vi "create_dataset.vi"() -> ()   [LabVIEW 2024]
uses:
  controls/class.ctl
  controls/cluster.ctl
  <vilib>/vision/Image Controls.llb/IMAQ Image.ctl
  <vilib>/vision/NI_Vision_Development_Module.lvlib
panel:
  in  "Redo":bool
  in  "Undo":bool
  in  "Stop":bool
  in  "Help":bool
  in  "Next":bool
  in  "Previous":bool
  out "Number of features:":dbl
  in  "Feature Type:":T1 items=["weld", "corrugation"]
  in  "Change Directory":bool
  out "Current Image name":string
  in  "Database Directory:":path=path "C:/Users/Naomi Tan/Documents/Gillette/FACE/02 - Code/FACE_software/images/test/ST100242_CAMFACE_LOCGLICR_RN3147_SHV3Post_POSleft.jpg"
  in  "Tab Control":enum32{"Setup", "Create"}(tab)
  in  "Dataset Directory:":path=path "C:/Users/J Gordon/Documents/Create Dataset/images"
  in  "Image Directory/File:":path=path "C:/Users/J Gordon/Documents/Create Dataset/images/test"
  in  "Start":bool
  out "of":i32
  out "Image":i32
  out "Image":T2(plugin-control)
  out "Zoom Window":T2(plugin-control)
  # "Create Custom\nDataset"
  # "Select Directories"
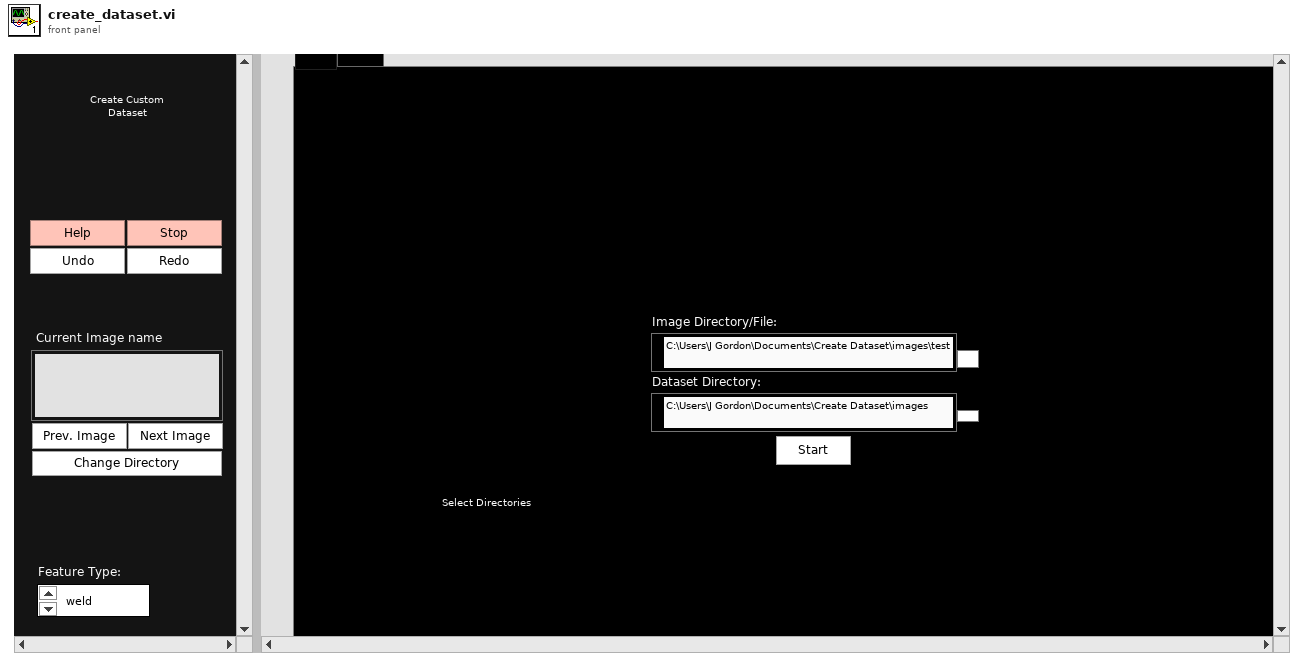
[diagram p1: front panel]
types:
  T1 = typedef "Class.ctl" = u16
  T2 = typedef "IMAQ Image.ctl" = refnum<image>
  T3 = enum8{"Enabled", "Disabled", "Disabled and Grayed Out"}
  T4 = cluster{"[0]":dbl, "[1]":dbl, "[2]":dbl, "[3]":dbl}[]
  T5 = typedef "cluster.ctl" = cluster{"Image path":path, "Image path array":path[], "Image index":u32, "Dataset Directory:":path, "Exists":bool, "classes":string[], "bboxes":cluster{"[0]":dbl, "[1]":dbl, "[2]":dbl, "[3]":dbl}[], "n":dbl, "Image":T2, "Image name":string, "classes history":string[], "bboxes":cluster{"[0]":dbl, "[1]":dbl, "[2]":dbl, "[3]":dbl}[], "Model Path:":path, "Classes Path:":path, "scores":dbl[], "Confidence":dbl}
  T6 = cluster{"[0]":i32, "[1]":i32, "[2]":i32, "[3]":i32}[]
  T7 = typedef "Image Type" = u32
  T8 = cluster{"Global Rectangle":i32[], "Contours":cluster{"Contour Type":u32, "ROI Type":u32, "Points":i32[]}[]}
  T9 = cluster{"Numeric Control":dbl, "Numeric Control":dbl, "width":dbl, "height":dbl}
  T10 = cluster{"Numeric Control":dbl, "Numeric Control":dbl, "width":dbl, "height":dbl}[]
  T11 = cluster{"[0]":dbl, "[1]":dbl, "[2]":dbl, "[3]":dbl}
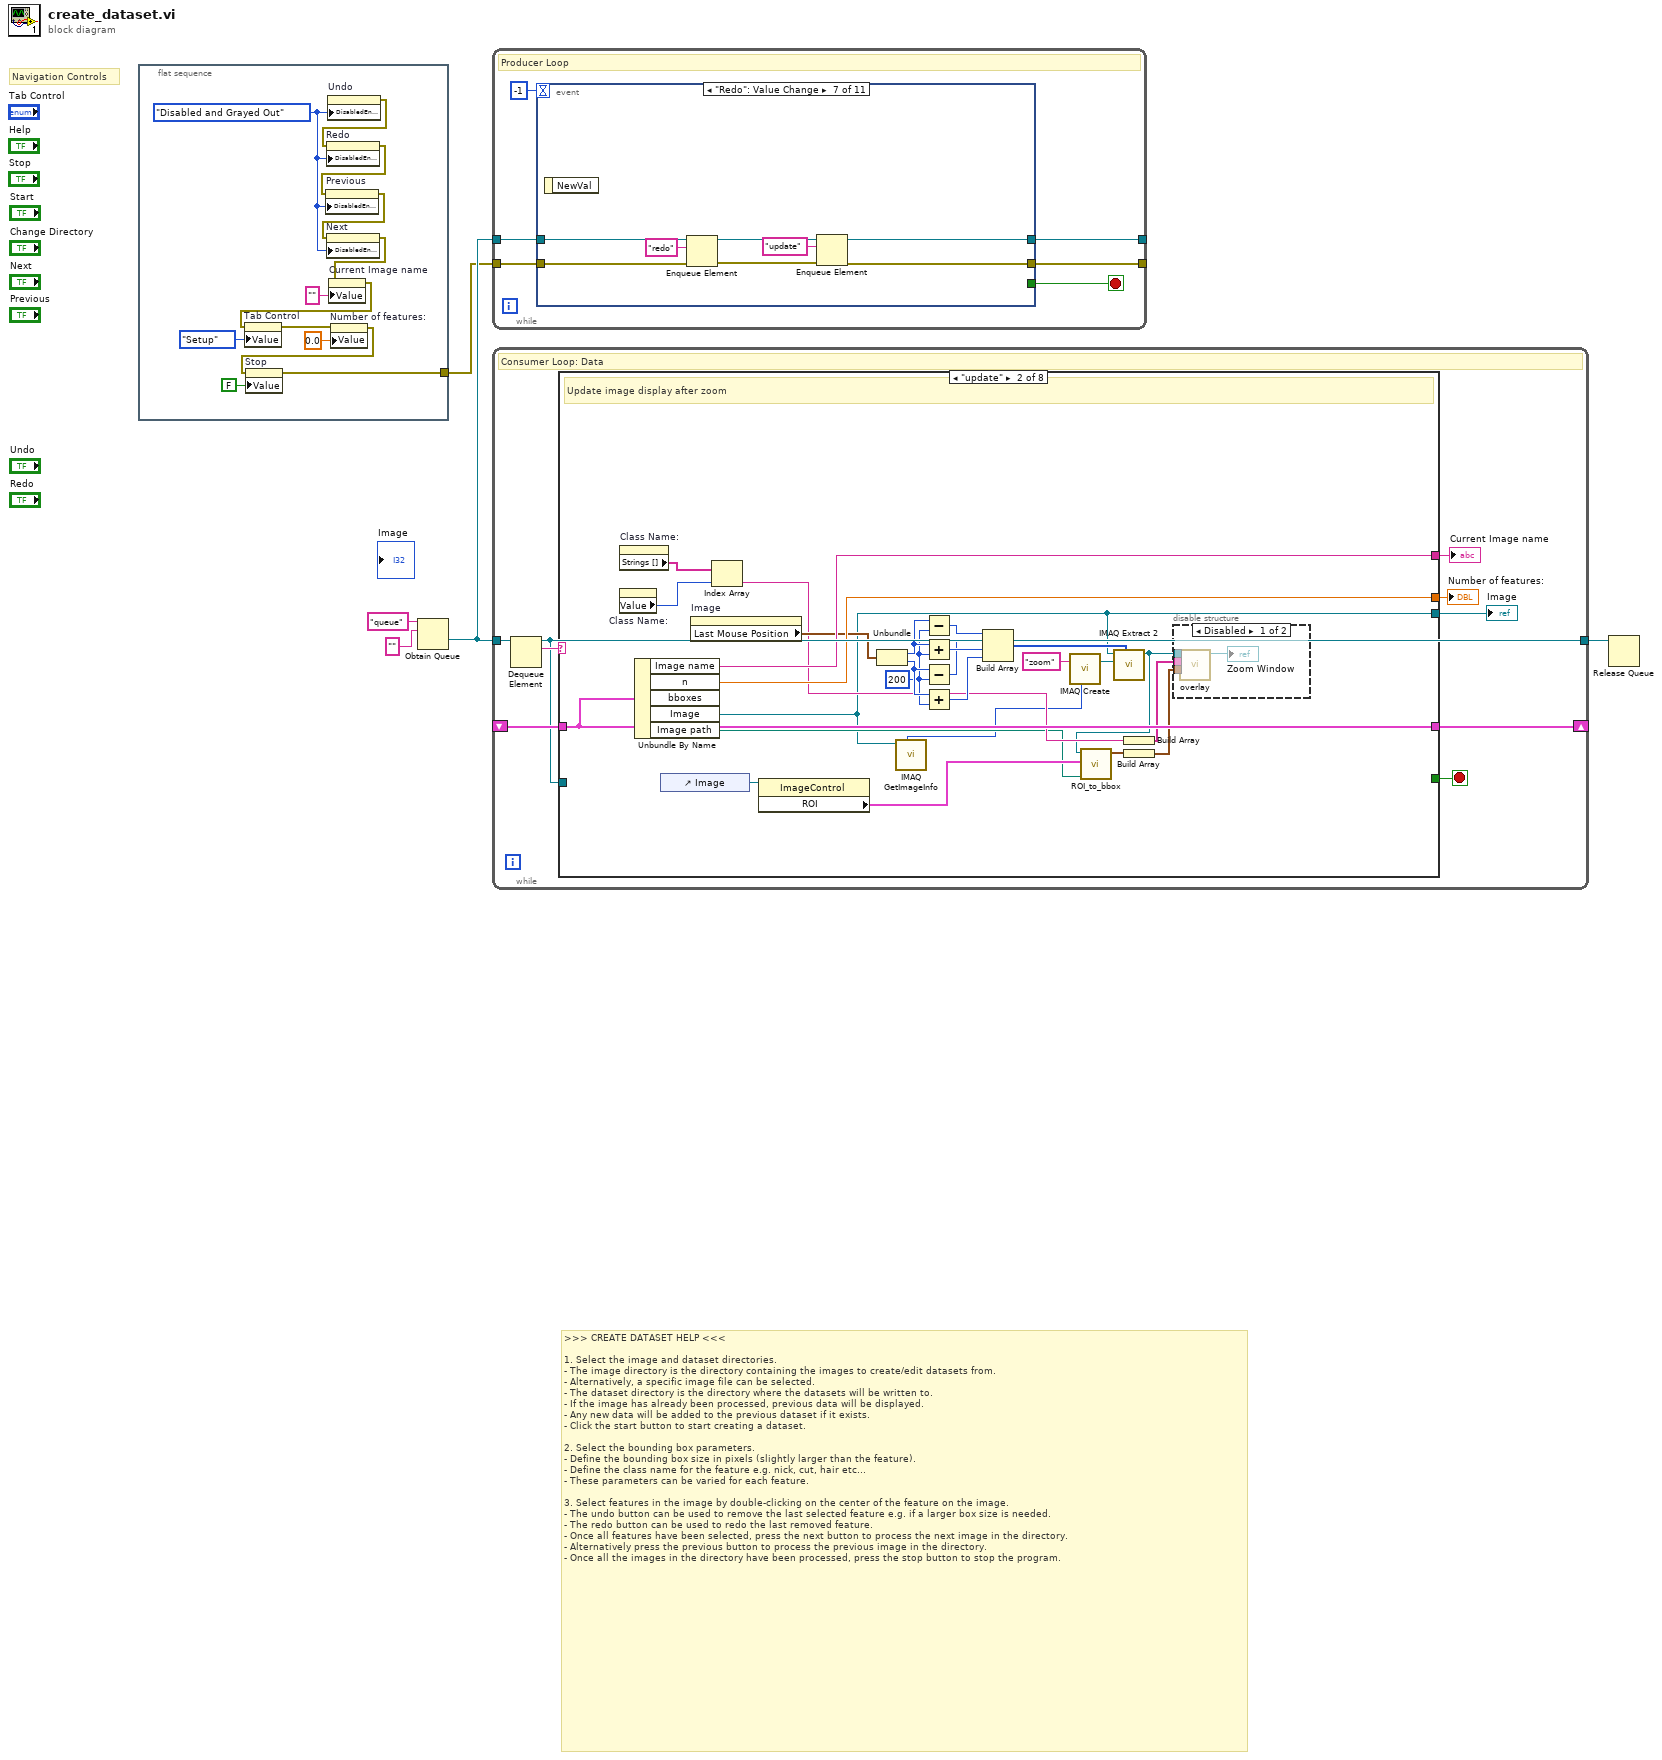
[diagram p0: block diagram]
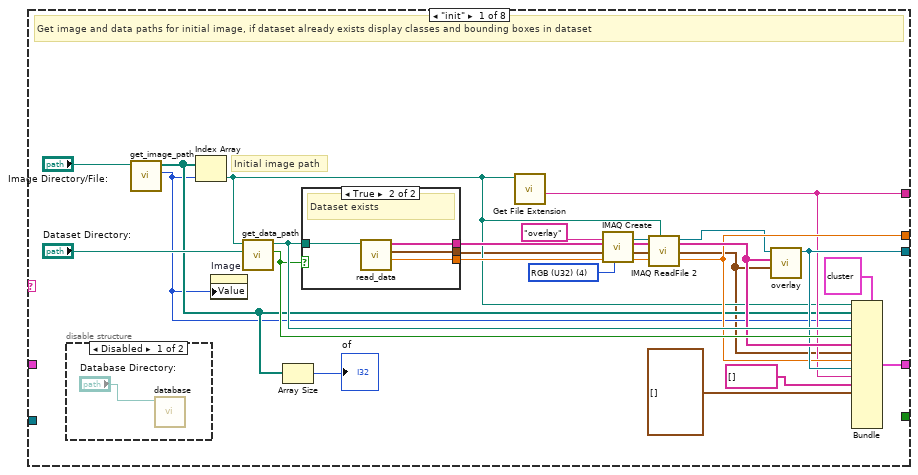
[diagram p2: hidden frame]
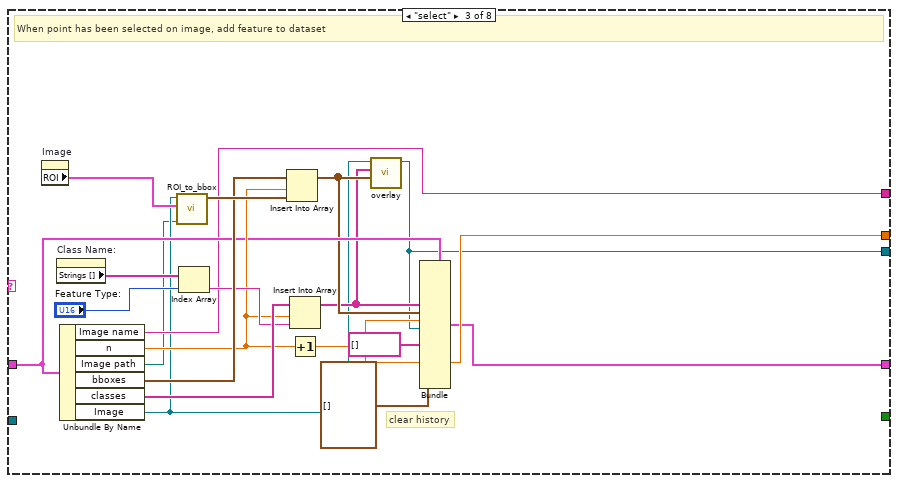
[diagram p6: hidden frame]
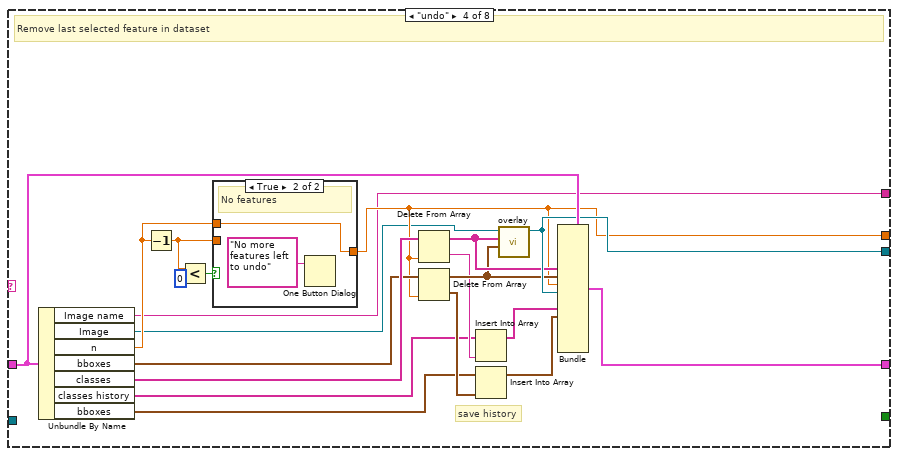
[diagram p7: hidden frame]
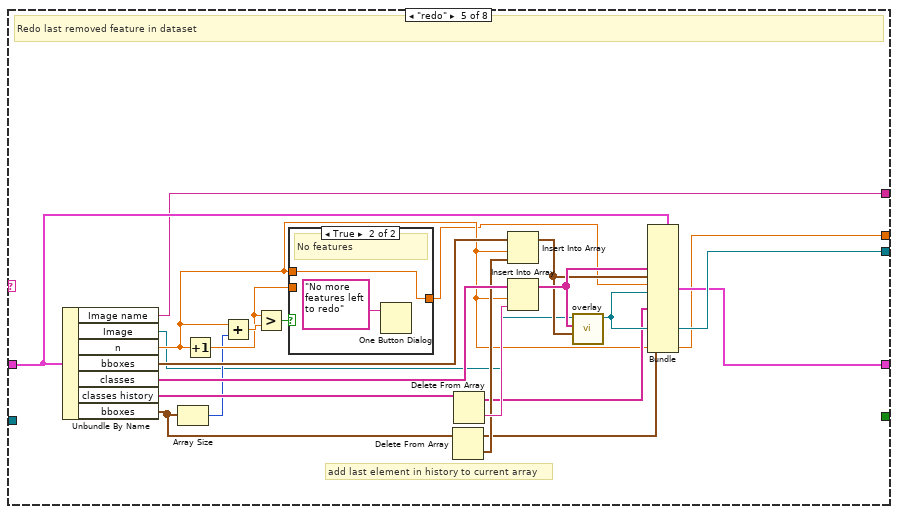
[diagram p9: hidden frame]
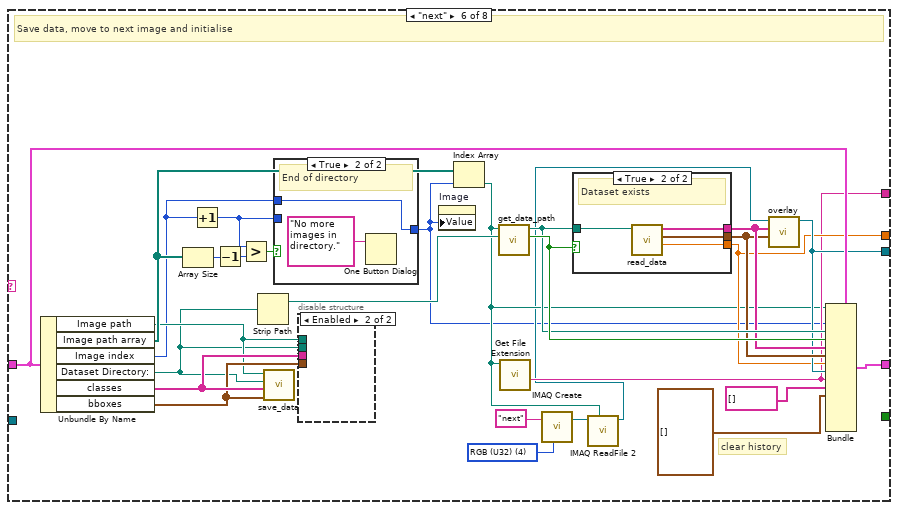
[diagram p11: hidden frame]
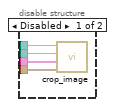
[diagram p12: hidden frame]
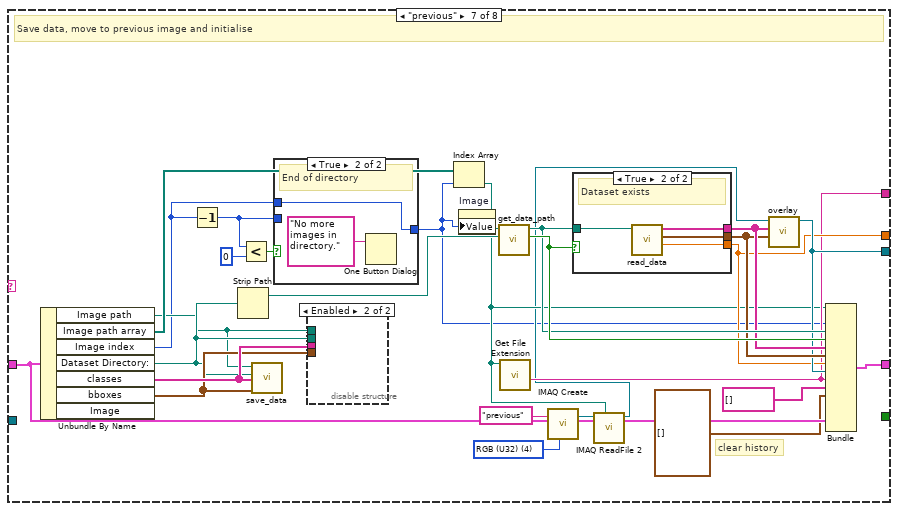
[diagram p15: hidden frame]
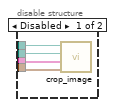
[diagram p16: hidden frame]
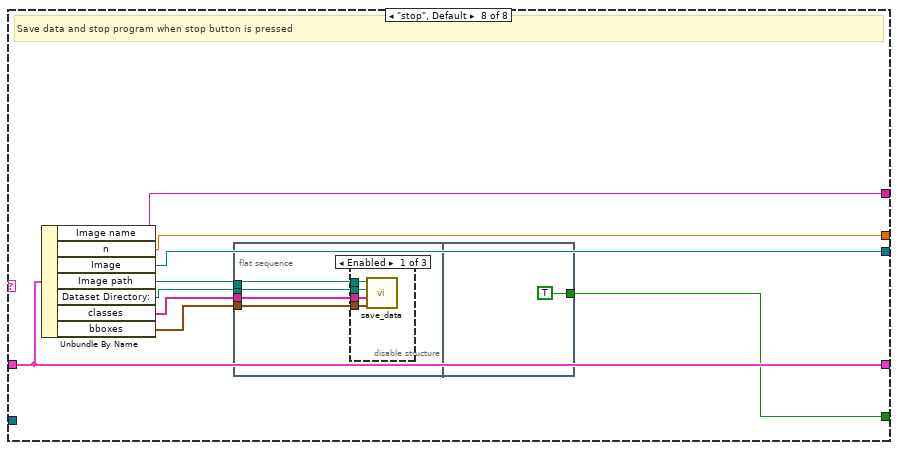
[diagram p19: hidden frame]
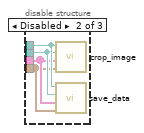
[diagram p20: hidden frame]
diagram:
  # ">>> CREATE DATASET HELP <<<\n\n1. Select the image and dataset directories.\n- The image directory is the directory containing the images to create/edit datasets from.\n- Alternatively, a specific image file can be selected.\n- The dataset directory is the directory where the datasets will be written to.\n- If the image has already been processed, previous data will be displayed.\n- Any new data will be added to the previous dataset if it exists.\n- Click the start button to start creating a dataset.\n\n2. Select the bounding box parameters.\n- Define the bounding box size in pixels (slightly larger than the feature).\n- Define the class name for the feature e.g. nick, cut, hair etc...\n- These parameters can be varied for each feature.\n\n3. Select features in the image by double-clicking on the center of the feature on the image.\n- The undo button can be used to remove the last selected feature e.g. if a larger box size is needed.\n- The redo button can be used to redo the last removed feature.\n- Once all features have been selected, press the next button to process the next image in the directory.\n- Alternatively press the previous button to process the previous image in the directory.\n- Once all the images in the directory have been processed, press the stop button to stop the program."
  # "Navigation Controls"
  n1 = flat-sequence {
    tunnel: [w6] -> w2
    frame #0 {
      w14 = T3."Disabled and Grayed Out" ("Disabled")
      n2 = property on="Undo" class="Bool"("DisabledEnum"=w14) -> (error out=w13:errorcluster)  [unwired: 2 in, 1 out]
      n3 = property on="Redo" class="Bool"(error in=w13, "DisabledEnum"=w14) -> (error out=w12:errorcluster)  [unwired: 1 in, 1 out]
      n4 = property on="Previous" class="Bool"(error in=w12, "DisabledEnum"=w14) -> (error out=w11:errorcluster)  [unwired: 1 in, 1 out]
      n5 = property on="Next" class="Bool"(error in=w11, "DisabledEnum"=w14) -> (error out=w10:errorcluster)  [unwired: 1 in, 1 out]
      n6 = property on="Current Image name" class="Str"(error in=w10, "Value"="" ("Image name:")) -> (error out=w9:errorcluster)  [unwired: 1 in, 1 out]
      n7 = property on="Tab Control" class="TabCtl (strict)"(error in=w9, "Value"=enum32{"Setup", "Create"}."Setup" ("Tab Control")) -> (error out=w8:errorcluster)  [unwired: 1 in, 1 out]
      n8 = property on="Number of features:" class="DigNum (strict)"(error in=w8, "Value"=0.0 ("Number of features:")) -> (error out=w7:errorcluster)  [unwired: 1 in, 1 out]
      n9 = property on="Stop" class="Bool (strict)"(error in=w7, "Value"=FALSE ("Stop Button")) -> (error out=w6:errorcluster)  [unwired: 1 in, 1 out]
    }
  }
  n10 = Obtain Queue(name (unnamed)="queue", element data type="" ("name (unnamed)")) -> (queue out=w3:refnum<queue>)  [unwired: 3 in, 2 out]
  n11 = while {
    tunnel: w3 -> [w23]
    tunnel: [w22] -> _
    tunnel: [w21] -> _
    tunnel: w2 -> [w20]
    stop <- w24 stop-if-true
    # "Producer Loop"
    n12 = event shown="[6] \"Redo\": Value Change" {
      selector: _ -> [_ _ _ _ _ _ _ _ _ _ _]
      dyn-events: _ -> [_ _ _ _ _ _ _ _ _ _ _]
      timeout: -1 -> [_ _ _ _ _ _ _ _ _ _ _]
      tunnel: w23 -> [w27 w33 w41 w59 w64 w99 w107 w114 w122 w125 w130]
      tunnel: [w27 w31 w42 w59 w63 w93 w103 w111 w120 w125 w129] -> w22
      tunnel: [_ TRUE _ _ _ _ _ _ _ _ _] -> w24
      tunnel: [w25 w29 w40 w56 w62 w92 w102 w109 w119 w124 w127] -> w21
      tunnel: w20 -> [w25 w28 w34 w56 w61 w97 w105 w108 w116 w124 w128]
      event "Help": Value Change {
        n13 = event-data() -> ()  [unwired: 1 in, 1 out]
        n14 = One Button Dialog(message="                                                                 >>> CREATE DATASET HELP <<<\n\n1. Select the image and dataset directories.\n- The image directory is the directory containing the images to create/edit datasets from.\n- Alternatively, a specific image file can be selected.\n- The dataset directory is the directory where the datasets will be written to.\n- If the image has already been processed, previous data will be displayed.\n- Any new data will be added to the previous dataset if it exists.\n- Click the start button to start creating a dataset.\n\n2. Select the bounding box parameters.\n- Define the bounding box size in pixels (slightly larger than the feature).\n- Define the class name for the feature e.g. nick, cut, hair etc...\n- These parameters can be varied for each feature.\n\n3. Select features in the image by double-clicking on the center of the feature on the image.\n- The undo button can be used to remove the last selected feature e.g. if a larger box size is needed.\n- The redo button can be used to redo the last removed feature.\n- Once all features have been selected, press the next button to process the next image in the directory.\n- Alternatively press the previous button to process the previous image in the directory.\n- Once all the images in the directory have been processed, press the stop button to stop the program.") -> ()  [unwired: 1 in, 1 out]
      }
      event "Stop": Value Change {
        n15 = event-data() -> ()  [unwired: 1 in, 1 out]
        n16 = Enqueue Element(queue=w33, element="stop" ("name (unnamed)"), error in (no error)=w28) -> (queue out=w31:refnum<queue>, error out=w29:errorcluster)  [unwired: 1 in, 1 out]
      }
      event "Start": Value Change {
        n17 = event-data() -> ()  [unwired: 1 in, 1 out]
        n18 = property on="Image Directory/File:" class="Path"() -> ("Value"=w36:path)  [unwired: 2 in, 2 out]
        n19 = property on="Dataset Directory:" class="Path"() -> ("Value"=w37:path)  [unwired: 2 in, 2 out]
        n20 = call <vilib>:"Check if File or Folder Exists.vi"("path"=w36) -> ("file or folder exists?"=w39:bool)  [unwired: 8 in, 2 out]
        n21 = call <vilib>:"Check if File or Folder Exists.vi"("path"=w37) -> ("file or folder exists?"=w38:bool)  [unwired: 8 in, 2 out]
        n22 = And(x=w39, y=w38) -> (x .and. y?=w35:bool)
        n23 = case shown="True" w35 {
          tunnel: [w45 w50] -> w42
          tunnel: w41 -> [w45 w54]
          tunnel: [w43 w47] -> w40
          tunnel: w34 -> [w43 w46]
          frame False {
            # "Directories don't exist"
            n24 = One Button Dialog(message="Image or dataset directory does not exist, please select another directory") -> ()  [unwired: 1 in, 1 out]
          }
          frame True {
            w52 = T3."Enabled" ("Disabled")
            # "Directories exist"
            n25 = Enqueue Element(queue=w54, element="init", error in (no error)=w46) -> (queue out=w49:refnum<queue>, error out=w48:errorcluster)  [unwired: 1 in, 1 out]
            n26 = property on="Tab Control" class="TabCtl (strict)"("Value"=enum32{"Setup", "Create"}."Create" ("Tab Control")) -> ()  [unwired: 2 in, 2 out]
            n27 = property on="Redo" class="Bool"("DisabledEnum"=w52) -> ()  [unwired: 2 in, 2 out]
            n28 = property on="Previous" class="Bool"("DisabledEnum"=w52) -> ()  [unwired: 2 in, 2 out]
            n29 = property on="Next" class="Bool"("DisabledEnum"=w52) -> ()  [unwired: 2 in, 2 out]
            n30 = Enqueue Element(queue=w49, element="update", error in (no error)=w48) -> (queue out=w50:refnum<queue>, error out=w47:errorcluster)  [unwired: 1 in, 1 out]
            n31 = property on="Undo" class="Bool"("DisabledEnum"=w52) -> ()  [unwired: 2 in, 2 out]
          }
        }
      }
      event "Change Directory": Value Change {
        w57 = T3."Disabled and Grayed Out" ("Disabled")
        n32 = event-data() -> ()  [unwired: 1 in, 1 out]
        n33 = property on="Tab Control" class="TabCtl (strict)"("Value"=enum32{"Setup", "Create"}."Setup" ("Tab Control")) -> ()  [unwired: 2 in, 2 out]
        n34 = property on="Undo" class="Bool"("DisabledEnum"=w57) -> ()  [unwired: 2 in, 2 out]
        n35 = property on="Redo" class="Bool"("DisabledEnum"=w57) -> ()  [unwired: 2 in, 2 out]
        n36 = property on="Previous" class="Bool"("DisabledEnum"=w57) -> ()  [unwired: 2 in, 2 out]
        n37 = property on="Next" class="Bool"("DisabledEnum"=w57) -> ()  [unwired: 2 in, 2 out]
      }
      event "Image": Mouse Up {
        n38 = event-data() -> ()  [unwired: 1 in, 1 out]
        n39 = disable-structure shown="Enabled" {
          disable-tunnel: w64 -> [w69 w84 _]
          disable-tunnel: [w68 w83 _] -> w63
          disable-tunnel: [w67 w82 _] -> w62
          disable-tunnel: TRUE ("Double Click") -> [w66 w81 _]
          disable-tunnel: w61 -> [w65 w80 _]
          frame Enabled {
            n40 = case shown="True" w66 {
              tunnel: w69 -> [w71 w78]
              tunnel: [w71 w74] -> w68
              tunnel: [w70 w72] -> w67
              tunnel: w65 -> [w70 w77]
              frame False {
              }
              frame True {
                n41 = Enqueue Element(queue=w78, element="select" ("name (unnamed)"), error in (no error)=w77) -> (queue out=w75:refnum<queue>, error out=w73:errorcluster)  [unwired: 1 in, 1 out]
                n42 = Enqueue Element(queue=w75, element="update" ("name (unnamed)"), error in (no error)=w73) -> (queue out=w74:refnum<queue>, error out=w72:errorcluster)  [unwired: 1 in, 1 out]
              }
            }
          }
          frame Disabled {
            n43 = case shown="True" w81 {
              tunnel: w84 -> [w86 w90]
              tunnel: [w86 w88] -> w83
              tunnel: [w85 w87] -> w82
              tunnel: w80 -> [w85 w89]
              frame False {
              }
              frame True {
                n44 = Enqueue Element(queue=w90, element="box" ("name (unnamed)"), error in (no error)=w89) -> (queue out=w88:refnum<queue>, error out=w87:errorcluster)  [unwired: 1 in, 1 out]
              }
            }
          }
          frame Disabled {
          }
        }
      }
      event "Undo": Value Change {
        n45 = event-data() -> ()  [unwired: 1 in, 1 out]
        n46 = Enqueue Element(queue=w99, element="undo", error in (no error)=w97) -> (queue out=w95:refnum<queue>, error out=w94:errorcluster)  [unwired: 1 in, 1 out]
        n47 = Enqueue Element(queue=w95, element="update", error in (no error)=w94) -> (queue out=w93:refnum<queue>, error out=w92:errorcluster)  [unwired: 1 in, 1 out]
      }
      event "Redo": Value Change {
        n48 = event-data() -> ()  [unwired: 1 in, 1 out]
        n49 = Enqueue Element(queue=w107, element="redo", error in (no error)=w105) -> (queue out=w100:refnum<queue>, error out=w101:errorcluster)  [unwired: 1 in, 1 out]
        n50 = Enqueue Element(queue=w100, element="update", error in (no error)=w101) -> (queue out=w103:refnum<queue>, error out=w102:errorcluster)  [unwired: 1 in, 1 out]
      }
      event "Next": Value Change {
        n51 = event-data() -> ()  [unwired: 1 in, 1 out]
        n52 = Enqueue Element(queue=w114, element="next", error in (no error)=w108) -> (queue out=w112:refnum<queue>, error out=w110:errorcluster)  [unwired: 1 in, 1 out]
        n53 = Enqueue Element(queue=w112, element="update", error in (no error)=w110) -> (queue out=w111:refnum<queue>, error out=w109:errorcluster)  [unwired: 1 in, 1 out]
      }
      event "Previous": Value Change {
        n54 = event-data() -> ()  [unwired: 1 in, 1 out]
        n55 = Enqueue Element(queue=w122, element="previous", error in (no error)=w116) -> (queue out=w117:refnum<queue>, error out=w118:errorcluster)  [unwired: 1 in, 1 out]
        n56 = Enqueue Element(queue=w117, element="update", error in (no error)=w118) -> (queue out=w120:refnum<queue>, error out=w119:errorcluster)  [unwired: 1 in, 1 out]
      }
      event Timeout {
        n57 = event-data() -> ()  [unwired: 1 in, 1 out]
      }
      event "Image": Mouse Move {
        n58 = event-data() -> ()  [unwired: 1 in, 5 out]
        n59 = Enqueue Element(queue=w130, element="update", error in (no error)=w128) -> (queue out=w129:refnum<queue>, error out=w127:errorcluster)  [unwired: 1 in, 1 out]
      }
    }
  }
  n60 = while {
    tunnel: w3 -> [w139]
    tunnel: [w131] -> w1
    shift-right: [w135] -> _
    shift-left: _ -> [w133]
    stop <- w137 stop-if-true
    # "Consumer Loop: Data"
    n61 = Dequeue Element(queue=w139) -> (queue out=w131:refnum<queue>, element=w138:string)  [unwired: 2 in, 2 out]
    n62 = case shown="\"update\"" w138 {
      tunnel: [w155 w191 w204 w224 w240 w277 w315 w343] -> w136
      tunnel: [_ _ _ _ _ _ _ w339] -> w137
      tunnel: [w156 w167 w202 w233 w257 w278 w316 w341] -> w132
      tunnel: [w157 w190 w203 w228 w252 w284 w324 w347] -> w135
      tunnel: [w154 w189 w200 w220 w251 w276 w314 w340] -> w134
      tunnel: w133 -> [_ w190 w207 w234 w258 w285 w325 w347]
      tunnel: w131 -> [_ _ _ _ _ _ _ _]
      frame "init" {
        w147 = T7 4 items=["Grayscale (U8)", "Grayscale (I16)", "Grayscale (SGL)", "Complex (CSG)", "RGB (U32)", "HSL (U32)", "RGB (U64)", "Grayscale (U16)"] ("Image Type")
        # "Initial image path"
        # "Get image and data paths for initial image, if dataset already exists display classes and bounding boxes in dataset"
        n63 = disable-structure shown="Disabled" {
          frame Disabled {
            n64 = call "database.vi"("db file"="Database Directory:") -> ()  [unwired: 9 in, 2 out]
          }
          frame Enabled {
          }
        }
        n65 = call "get_image_path.vi"("Image directory/path"="Image Directory/File:") -> ("Init image index"=w142:u32, "Image path array"=w144:path[])  [unwired: 9 in]
        n66 = Index Array(array=w144, index=w142) -> (element=w146:path)
        n67 = property on="Image" class="DigNum (strict)"("Value"=w142) -> ()  [unwired: 2 in, 2 out]
        n68 = call "get_data_path.vi"("Dataset directory"="Dataset Directory:", "Image path"=w146) -> ("Exists"=w159:bool, "Dataset path"=w160:path)  [unwired: 8 in]
        n69 = Array Size(array=w144) -> (size(s)=→"of":i32)
        n70 = case shown="True" w159 {
          tunnel: w160 -> [_ w162]
          tunnel: [_ w165] -> w141
          tunnel: [_ w164] -> w155
          tunnel: [_ w163] -> w158
          frame False {
            # "Dataset doesn't exist"
          }
          frame True {
            # "Dataset exists"
            n71 = call "read_data.vi"("Data path"=w162) -> ("n"=w164:dbl, "bboxes"=w165:T4, "classes"=w163:string[])  [unwired: 7 in, 1 out]
          }
        }
        n72 = call <vilib>:"Get File Extension.vi"("file"=w146) -> ("filename without extension"=w154:string)  [unwired: 6 in, 4 out]
        n73 = call "IMAQ Create"("Image Name"="overlay", "Image Type"=w147) -> ("New Image"=w148:T2)  [unwired: 3 in, 1 out]
        n74 = call "IMAQ ReadFile 2"("File Path"=w146, "Image"=w148) -> ("Image Out"=w145:T2)  [unwired: 5 in, 4 out]
        n75 = call "overlay.vi"("Image in"=w145, "classes"=w158, "bboxes"=w141) -> ("Image"=w156:T2)  [unwired: 7 in]
        n76 = Bundle(cluster=T5 {"Image path"=path "", "Image path array"=[], "Image index"=0, "Dataset Directory:"=path "", "Exists"=FALSE, "classes"=[], "bboxes"=[], "n"=0.0, "Image"=refnum, "Image name"="", "classes history"=[], "bboxes"=[], "Model Path:"=path "", "Classes Path:"=path "", "scores"=[], "Confidence"=0.0}, "Image path"=w146, "Image path array"=w144, "Image index"=w142, "Dataset Directory:"=w160, "Exists"=w159, "classes"=w158, "bboxes"=w141, "n"=w155, "Image"=w156, "Image name"=w154, "classes history"=string[] [], "bboxes"=T4 []) -> (w157:T5)  [unwired: 4 in]
      }
      frame "update" {
        w180 = 200 ("y")
        # "Update image display after zoom"
        n77 = property on="Class Name:" class="Ring (strict)"() -> ("Strings []"=w175:string[])  [unwired: 2 in, 2 out]
        n78 = property on="Class Name:" class="Ring (strict)"() -> ("Value"=w176:T1)  [unwired: 2 in, 2 out]
        n79 = Unbundle By Name(w190) -> ("Image name"=w189:string, "n"=w191:dbl, "Image"=w167:T2, "Image path"=w168:path)  [unwired: 1 out]
        n80 = control-ref of="Image"() -> (w170:refnum<vi>)
        n81 = property on="Image" class="ImageControl"() -> ("Last Mouse Position"=w185:cluster{"X":i32, "Y":i32})  [unwired: 2 in, 2 out]
        n82 = Index Array(array=w175, index=w176) -> (element=w173:string)
        n83 = property class="ImageControl"(reference=w170) -> ("ROI"=w169:T8)  [unwired: 1 in, 2 out]
        n84 = Unbundle(w185) -> ("X"=w182:i32, "Y"=w181:i32)
        n85 = call "IMAQ GetImageInfo"("Image"=w167) -> ("Image Type"=w166:T7)  [unwired: 3 in, 7 out]
        n86 = Subtract(x=w182, y=w180) -> (x-y=w179:i32)
        n87 = Add(x=w182, y=w180) -> (x+y=w186:i32)
        n88 = Subtract(x=w181, y=w180) -> (x-y=w178:i32)
        n89 = Add(x=w181, y=w180) -> (x+y=w187:i32)
        n90 = Build Array(w179, w178, w186, w187) -> (w188:i32[])
        n91 = call "IMAQ Create"("Image Name"="zoom", "Image Type"=w166) -> ("New Image"=w184:T2)  [unwired: 3 in, 1 out]
        n92 = call "IMAQ Extract 2"("Optional Rectangle"=w188, "Image Dst"=w184, "Image Src"=w167) -> ("Image Dst Out"=w171:T2)  [unwired: 7 in, 1 out]
        n93 = call "ROI_to_bbox.vi"("Image path"=w168, "ROI"=w169, "Image in"=w171) -> ("bbox"=w174:T9)  [unwired: 8 in]
        n94 = Build Array(w173) -> (w172:string[])
        n95 = Build Array(w174) -> (w177:T10)
        n96 = disable-structure shown="Disabled" {
          disable-tunnel: w177 -> [w195 _]
          disable-tunnel: w172 -> [w194 _]
          disable-tunnel: w171 -> [w192 _]
          frame Disabled {
            n97 = call "overlay.vi"("Image in"=w192, "classes"=w194, "bboxes"=w195) -> ("Image"=→"Zoom Window":T2)  [unwired: 7 in]
          }
          frame Enabled {
          }
        }
      }
      frame "select" {
        # "clear history"
        # "When point has been selected on image, add feature to dataset"
        n98 = property on="Image" class="ImageControl"() -> ("ROI"=w214:T8)  [unwired: 2 in, 2 out]
        n99 = property on="Class Name:" class="Ring (strict)"() -> ("Strings []"=w212:string[])  [unwired: 2 in, 2 out]
        n100 = Unbundle By Name(w207) -> ("Image name"=w200:string, "n"=w208:dbl, "Image path"=w196:path, "bboxes"=w211:T4, "classes"=w210:string[], "Image"=w197:T2)
        n101 = call "ROI_to_bbox.vi"("Image path"=w196, "ROI"=w214, "Image in"=w197) -> ("bbox"=w213:T9)  [unwired: 8 in]
        n102 = Index Array(array=w212, index="Feature Type:") -> (element=w209:string)
        n103 = Insert Into Array(array=w211, index=w208, new element=w213) -> (w206:T4)
        n104 = Insert Into Array(array=w210, index=w208, new element=w209) -> (w205:string[])
        n105 = Increment(x=w208) -> (x+1=w204:dbl)
        n106 = call "overlay.vi"("Image in"=w197, "classes"=w205, "bboxes"=w206) -> ("Image"=w202:T2)  [unwired: 7 in]
        n107 = Bundle(cluster=w207, "classes"=w205, "bboxes"=w206, "n"=w204, "Image"=w202, "classes history"=string[] [], "bboxes"=T6 [] ("bboxes history")) -> (w203:T5)  [unwired: 10 in]
      }
      frame "undo" {
        # "save history"
        # "Remove last selected feature in dataset"
        n108 = Unbundle By Name(w234) -> ("Image name"=w220:string, "Image"=w215:T2, "n"=w221:dbl, "bboxes"=w231:T4, "classes"=w232:string[], "classes history"=w219:string[], "bboxes"=w218:T4)
        n109 = Decrement(x=w221) -> (x-1=w226:dbl)
        n110 = Less?(x=w226, y=u32 0) -> (x < y?=w227:bool)
        n111 = case shown="True" w227 {
          tunnel: w226 -> [w235 _]
          tunnel: [w235 w236] -> w224
          tunnel: w221 -> [_ w236]
          frame False {
            # "Index in range"
          }
          frame True {
            # "No features"
            n112 = One Button Dialog(message="No more features left to undo") -> ()  [unwired: 1 in, 1 out]
          }
        }
        n113 = Delete From Array(array=w232, index=w224) -> (deleted portion=w223:string, array with subset deleted=w230:string[])  [unwired: 1 in]
        n114 = Delete From Array(array=w231, index=w224) -> (deleted portion=w222:T11, array with subset deleted=w229:T4)  [unwired: 1 in]
        n115 = Insert Into Array(array=w219, new element=w223) -> (w217:string[])  [unwired: 1 in]
        n116 = Insert Into Array(array=w218, new element=w222) -> (w216:T4)  [unwired: 1 in]
        n117 = call "overlay.vi"("Image in"=w215, "classes"=w230, "bboxes"=w229) -> ("Image"=w233:T2)  [unwired: 7 in]
        n118 = Bundle(cluster=w234, "classes"=w230, "bboxes"=w229, "n"=w224, "Image"=w233, "classes history"=w217, "bboxes"=w216) -> (w228:T5)  [unwired: 10 in]
      }
      frame "redo" {
        # "add last element in history to current array"
        # "Redo last removed feature in dataset"
        n119 = Unbundle By Name(w258) -> ("Image name"=w251:string, "Image"=w238:T2, "n"=w240:dbl, "bboxes"=w255:T4, "classes"=w256:string[], "classes history"=w250:string[], "bboxes"=w242:T4)
        n120 = Array Size(array=w242) -> (size(s)=w241:i32)
        n121 = Increment(x=w240) -> (x+1=w243:dbl)
        n122 = Add(x=w240, y=w241) -> (x+y=w245:dbl)
        n123 = Greater?(x=w243, y=w245) -> (0:w244:bool)
        n124 = case shown="True" w244 {
          tunnel: w243 -> [w259 _]
          tunnel: [w259 w260] -> w239
          tunnel: w240 -> [_ w260]
          frame False {
            # "Index in range"
          }
          frame True {
            # "No features"
            n125 = One Button Dialog(message="No more features left to redo") -> ()  [unwired: 1 in, 1 out]
          }
        }
        n126 = Delete From Array(array=w242) -> (deleted portion=w248:T11, array with subset deleted=w246:T4)  [unwired: 2 in]
        n127 = Delete From Array(array=w250) -> (deleted portion=w249:string, array with subset deleted=w247:string[])  [unwired: 2 in]
        n128 = Insert Into Array(array=w255, index=w240, new element=w248) -> (w253:T4)
        n129 = Insert Into Array(array=w256, index=w240, new element=w249) -> (w254:string[])
        n130 = call "overlay.vi"("Image in"=w238, "classes"=w254, "bboxes"=w253) -> ("Image"=w257:T2)  [unwired: 7 in]
        n131 = Bundle(cluster=w258, "classes"=w254, "bboxes"=w253, "n"=w239, "Image"=w257, "classes history"=w247, "bboxes"=w246) -> (w252:T5)  [unwired: 10 in]
      }
      frame "next" {
        w267 = T7 4 items=["Grayscale (U8)", "Grayscale (I16)", "Grayscale (SGL)", "Complex (CSG)", "RGB (U32)", "HSL (U32)", "RGB (U64)", "Grayscale (U16)"] ("Image Type")
        # "clear history"
        # "Save data, move to next image and initialise"
        n132 = Unbundle By Name(w285) -> ("Image path"=w272:path, "Image path array"=w275:path[], "Image index"=w271:u32, "Dataset Directory:"=w262:path, "classes"=w274:string[], "bboxes"=w273:T4)
        n133 = Array Size(array=w275) -> (size(s)=w289:i32)
        n134 = Increment(x=w271) -> (x+1=w286:u32)
        n135 = Decrement(x=w289) -> (x-1=w288:i32)
        n136 = Greater?(x=w286, y=w288) -> (0:w287:bool)
        n137 = Strip Path(path=w262) -> (stripped path=w283:path)  [unwired: 1 out]
        n138 = call "save_data.vi"("bboxes"=w273, "classes"=w274, "Dataset path"=w262, "Image path"=w272) -> ()  [unwired: 8 in]
        n139 = case shown="True" w287 {
          tunnel: w286 -> [w298 _]
          tunnel: [w298 w299] -> w263
          tunnel: w271 -> [_ w299]
          frame False {
            # "Index in range"
          }
          frame True {
            # "End of directory"
            n140 = One Button Dialog(message="No more images in directory.") -> ()  [unwired: 1 in, 1 out]
          }
        }
        n141 = disable-structure shown="Enabled" {
          disable-tunnel: w262 -> [w293 _]
          disable-tunnel: w274 -> [w291 _]
          disable-tunnel: w273 -> [w292 _]
          disable-tunnel: w272 -> [w290 _]
          frame Disabled {
            n142 = call "crop_image.vi"("bboxes"=w292, "classes"=w291, "Dataset path"=w293, "Image path"=w290) -> ()  [unwired: 8 in]
          }
          frame Enabled {
          }
        }
        n143 = property on="Image" class="DigNum (strict)"("Value"=w263) -> ()  [unwired: 2 in, 2 out]
        n144 = Index Array(array=w275, index=w263) -> (element=w265:path)
        n145 = call "get_data_path.vi"("Dataset directory"=w283, "Image path"=w265) -> ("Exists"=w282:bool, "Dataset path"=w281:path)  [unwired: 8 in]
        n146 = call <vilib>:"Get File Extension.vi"("file"=w265) -> ("filename without extension"=w276:string)  [unwired: 6 in, 4 out]
        n147 = call "IMAQ Create"("Image Name"="next", "Image Type"=w267) -> ("New Image"=w268:T2)  [unwired: 3 in, 1 out]
        n148 = case shown="True" w282 {
          tunnel: w281 -> [_ w294]
          tunnel: [_ w297] -> w279
          tunnel: [_ w296] -> w277
          tunnel: [_ w295] -> w280
          frame False {
            # "Dataset doesn't exist"
          }
          frame True {
            # "Dataset exists"
            n149 = call "read_data.vi"("Data path"=w294) -> ("n"=w296:dbl, "bboxes"=w297:T4, "classes"=w295:string[])  [unwired: 7 in, 1 out]
          }
        }
        n150 = call "IMAQ ReadFile 2"("File Path"=w265, "Image"=w268) -> ("Image Out"=w264:T2)  [unwired: 5 in, 4 out]
        n151 = call "overlay.vi"("Image in"=w264, "classes"=w280, "bboxes"=w279) -> ("Image"=w278:T2)  [unwired: 7 in]
        n152 = Bundle(cluster=w285, "Image path"=w265, "Image index"=w263, "Dataset Directory:"=w281, "Exists"=w282, "classes"=w280, "bboxes"=w279, "n"=w277, "Image"=w278, "Image name"=w276, "classes history"=string[] [], "bboxes"=T6 []) -> (w284:T5)  [unwired: 5 in]
      }
      frame "previous" {
        w305 = T7 4 items=["Grayscale (U8)", "Grayscale (I16)", "Grayscale (SGL)", "Complex (CSG)", "RGB (U32)", "HSL (U32)", "RGB (U64)", "Grayscale (U16)"] ("Image Type")
        # "clear history"
        # "Save data, move to previous image and initialise"
        n153 = Unbundle By Name(w325) -> ("Image path"=w310:path, "Image path array"=w311:path[], "Image index"=w309:u32, "Dataset Directory:"=w312:path, "classes"=w323:string[], "bboxes"=w322:T4)  [unwired: 1 out]
        n154 = Decrement(x=w309) -> (x-1=w326:u32)
        n155 = Strip Path(path=w312) -> (stripped path=w321:path)  [unwired: 1 out]
        n156 = Less?(x=w326, y=u32 0) -> (x < y?=w327:bool)
        n157 = call "save_data.vi"("bboxes"=w322, "classes"=w323, "Dataset path"=w312, "Image path"=w310) -> ()  [unwired: 8 in]
        n158 = case shown="True" w327 {
          tunnel: w326 -> [w336 _]
          tunnel: [w336 w337] -> w301
          tunnel: w309 -> [_ w337]
          frame False {
            # "Index in range"
          }
          frame True {
            # "End of directory"
            n159 = One Button Dialog(message="No more images in directory.") -> ()  [unwired: 1 in, 1 out]
          }
        }
        n160 = disable-structure shown="Enabled" {
          disable-tunnel: w323 -> [w329 _]
          disable-tunnel: w322 -> [w328 _]
          disable-tunnel: w312 -> [w330 _]
          disable-tunnel: w310 -> [w331 _]
          frame Disabled {
            n161 = call "crop_image.vi"("bboxes"=w328, "classes"=w329, "Dataset path"=w330, "Image path"=w331) -> ()  [unwired: 8 in]
          }
          frame Enabled {
          }
        }
        n162 = Index Array(array=w311, index=w301) -> (element=w303:path)
        n163 = property on="Image" class="DigNum (strict)"("Value"=w301) -> ()  [unwired: 2 in, 2 out]
        n164 = call "get_data_path.vi"("Dataset directory"=w321, "Image path"=w303) -> ("Exists"=w320:bool, "Dataset path"=w319:path)  [unwired: 8 in]
        n165 = call <vilib>:"Get File Extension.vi"("file"=w303) -> ("filename without extension"=w314:string)  [unwired: 6 in, 4 out]
        n166 = call "IMAQ Create"("Image Name"="previous", "Image Type"=w305) -> ("New Image"=w306:T2)  [unwired: 3 in, 1 out]
        n167 = case shown="True" w320 {
          tunnel: w319 -> [_ w332]
          tunnel: [_ w335] -> w317
          tunnel: [_ w334] -> w315
          tunnel: [_ w333] -> w318
          frame False {
            # "Dataset doesn't exist"
          }
          frame True {
            # "Dataset exists"
            n168 = call "read_data.vi"("Data path"=w332) -> ("n"=w334:dbl, "bboxes"=w335:T4, "classes"=w333:string[])  [unwired: 7 in, 1 out]
          }
        }
        n169 = call "IMAQ ReadFile 2"("File Path"=w303, "Image"=w306) -> ("Image Out"=w302:T2)  [unwired: 5 in, 4 out]
        n170 = call "overlay.vi"("Image in"=w302, "classes"=w318, "bboxes"=w317) -> ("Image"=w316:T2)  [unwired: 7 in]
        n171 = Bundle(cluster=w325, "Image path"=w303, "Image index"=w301, "Dataset Directory:"=w319, "Exists"=w320, "classes"=w318, "bboxes"=w317, "n"=w315, "Image"=w316, "Image name"=w314, "classes history"=string[] [], "bboxes"=T6 []) -> (w324:T5)  [unwired: 5 in]
      }
      frame "stop", Default {
        # "Save data and stop program when stop button is pressed"
        n172 = Unbundle By Name(w347) -> ("Image name"=w340:string, "n"=w343:dbl, "Image"=w341:T2, "Image path"=w342:path, "Dataset Directory:"=w346:path, "classes"=w345:string[], "bboxes"=w344:T4)
        n173 = flat-sequence {
          tunnel: w346 -> [w351]
          tunnel: w345 -> [w350]
          tunnel: w344 -> [w349]
          tunnel: w342 -> [w348]
          tunnel: [TRUE] -> w339
          frame #0 {
            n174 = disable-structure shown="Enabled" {
              disable-tunnel: w351 -> [w355 w358 _]
              disable-tunnel: w350 -> [w354 w357 _]
              disable-tunnel: w349 -> [w353 w356 _]
              disable-tunnel: w348 -> [w352 w359 _]
              frame Enabled {
                n175 = call "save_data.vi"("bboxes"=w353, "classes"=w354, "Dataset path"=w355, "Image path"=w352) -> ()  [unwired: 8 in]
              }
              frame Disabled {
                n176 = call "crop_image.vi"("bboxes"=w356, "classes"=w357, "Dataset path"=w358, "Image path"=w359) -> ()  [unwired: 8 in]
                n177 = call "save_data.vi"("bboxes"=w356, "classes"=w357, "Dataset path"=w358, "Image path"=w359) -> ()  [unwired: 8 in]
              }
              frame Disabled {
              }
            }
          }
          frame #1 {
          }
        }
      }
    }
    "Image" <- w132
    "Number of features:" <- w136
    "Current Image name" <- w134
  }
  n178 = Release Queue(queue=w1) -> ()  [unwired: 2 in, 3 out]
